vi "EventListener.vi"() -> ()   [LabVIEW 2009]
uses:
  <vilib>/lvdsc/NI_DSC.lvlib
panel:
  in  "TERMINATE MEASUREMENT":bool
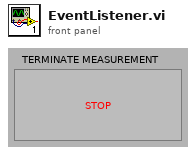
[diagram p1: front panel]
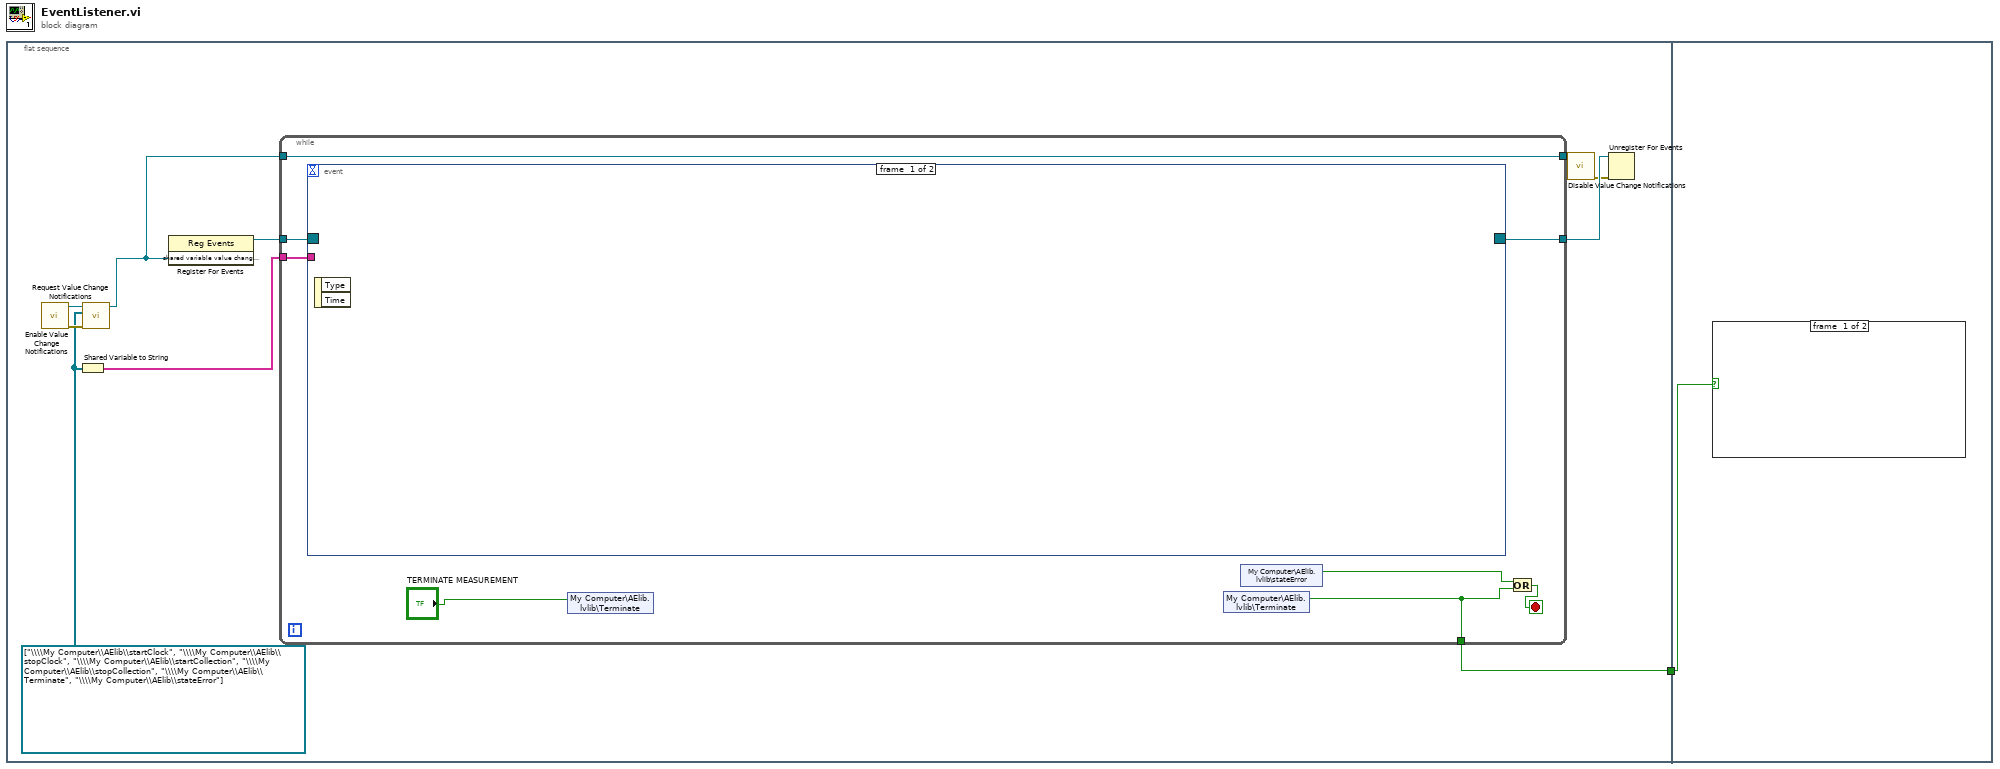
[diagram p0: block diagram]
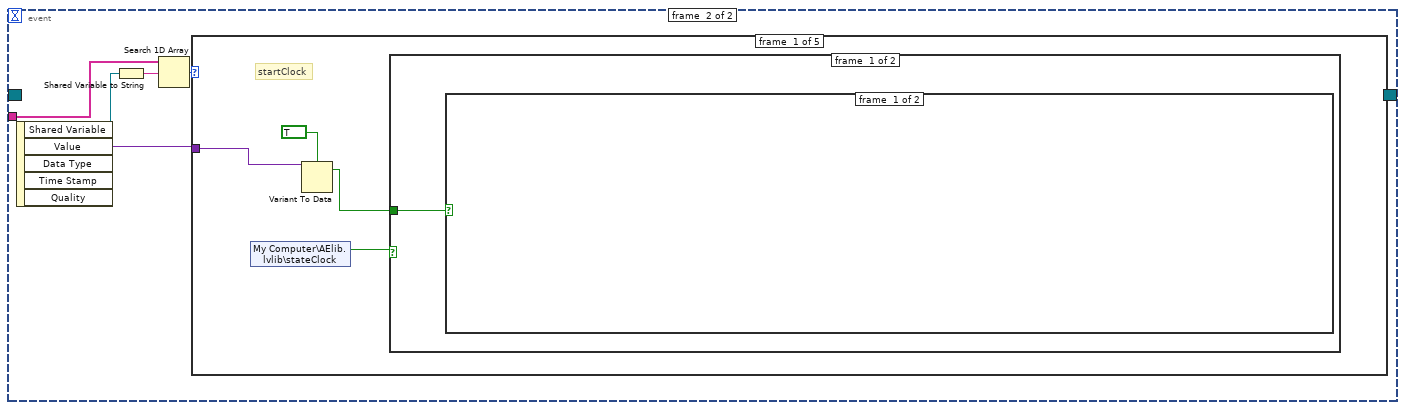
[diagram p2: hidden frame]
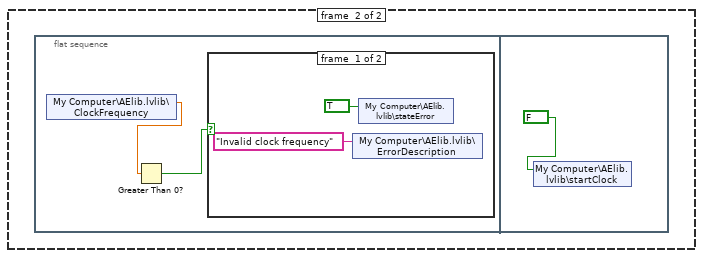
[diagram p3: hidden frame]
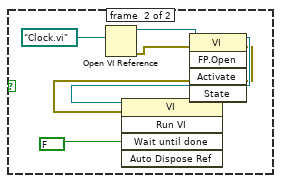
[diagram p4: hidden frame]
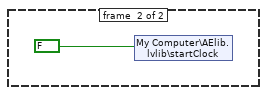
[diagram p6: hidden frame]
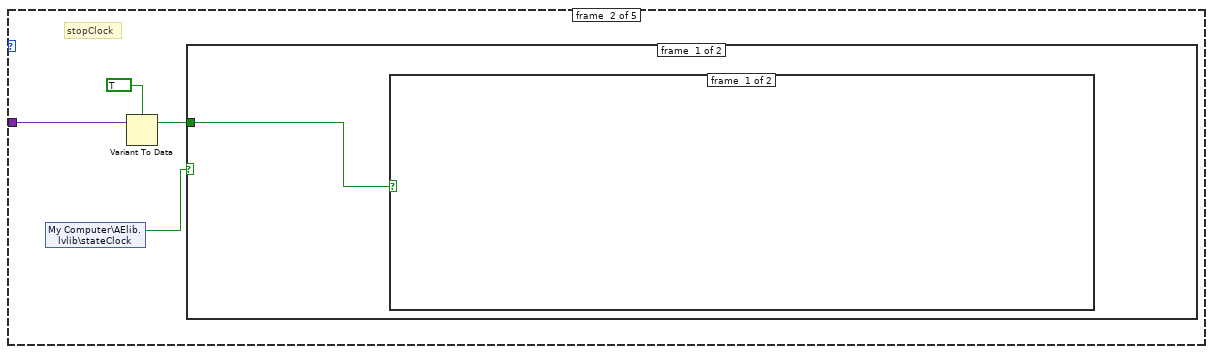
[diagram p7: hidden frame]
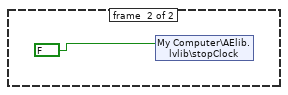
[diagram p8: hidden frame]
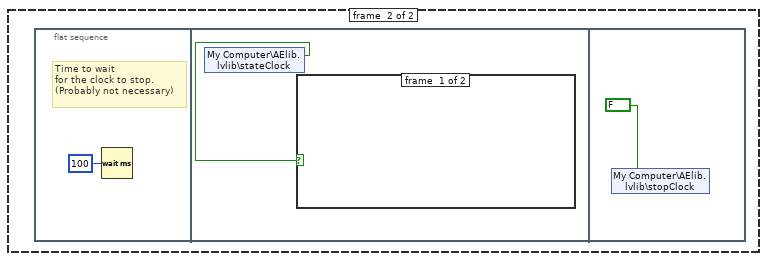
[diagram p10: hidden frame]
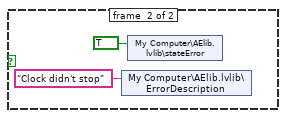
[diagram p11: hidden frame]
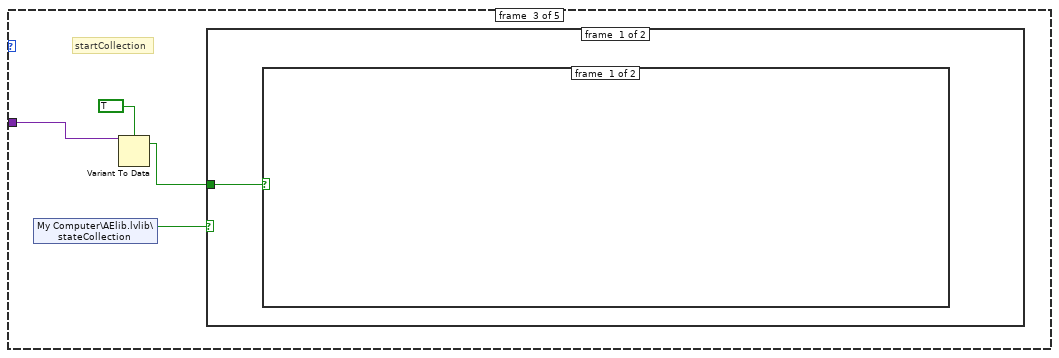
[diagram p12: hidden frame]
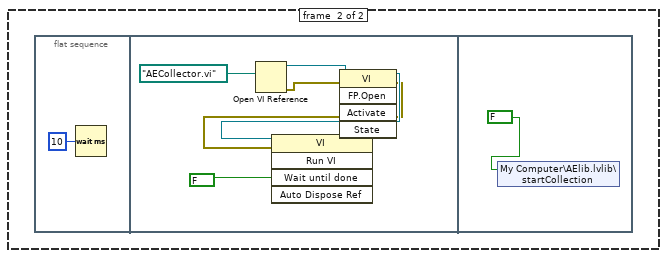
[diagram p13: hidden frame]
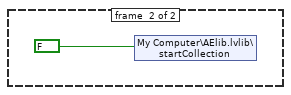
[diagram p15: hidden frame]
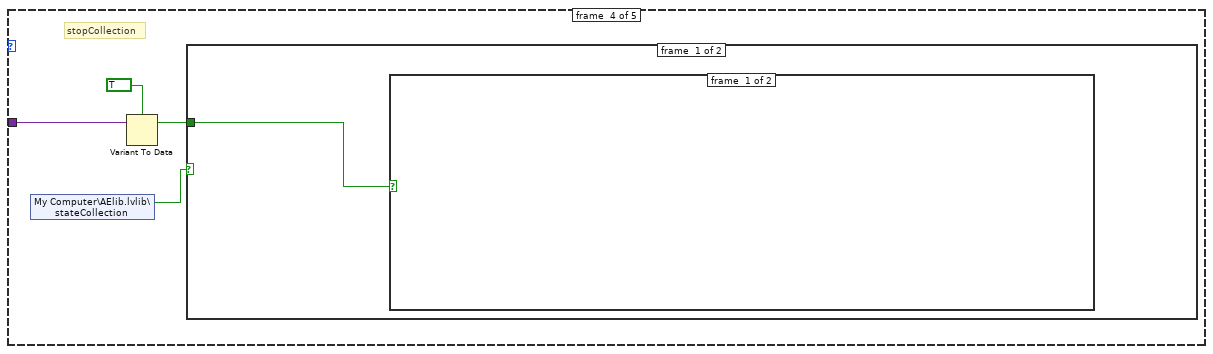
[diagram p16: hidden frame]
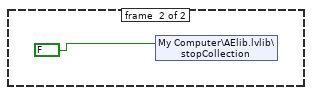
[diagram p17: hidden frame]
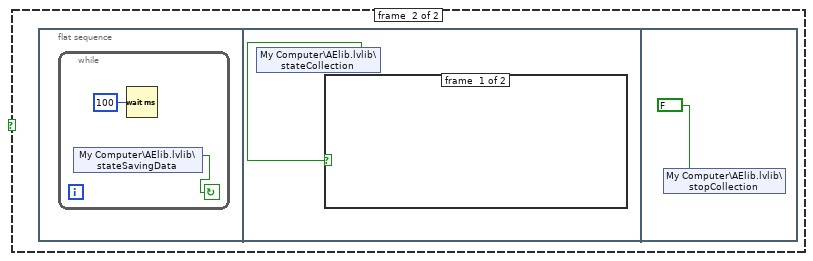
[diagram p19: hidden frame]
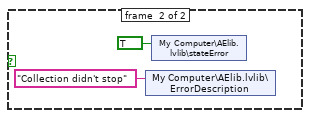
[diagram p20: hidden frame]
diagram:
  n1 = flat-sequence {
    tunnel: [w2] -> w1
    tunnel: w1 -> [w83]
    frame #0 {
      w4 = refnum<k21>[] ["\\\\My Computer\\AElib\\startClock", "\\\\My Computer\\AElib\\stopClock", "\\\\My Computer\\AElib\\startCollection", "\\\\My Computer\\AElib\\stopCollection", "\\\\My Computer\\AElib\\Terminate", "\\\\My Computer\\AElib\\stateError"] ("shared variables")
      n2 = call <vilib>:"Enable Value Change Notifications.vi"() -> ("error out"=w11:errorcluster, "shared variable value change notification"=w10:refnum<user-event>)  [unwired: 10 in]
      n3 = Shared Variable to String(1:w4) -> (0:w3:string[])
      n4 = call <vilib>:"Request Value Change Notifications.vi"("error in (no error)"=w11, "shared variables"=w4, "notification refnum"=w10) -> ("shared variable value change notification"=w8:refnum<user-event>)  [unwired: 6 in, 2 out]
      n5 = register-events(w8) -> (reference out=w9:refnum<event-registration>)  [unwired: 2 in, 1 out]
      n6 = while {
        tunnel: w9 -> [w19]
        tunnel: w8 -> [w18]
        tunnel: [w18] -> w7
        tunnel: [w17] -> w6
        tunnel: w3 -> [w16]
        tunnel: [w13] -> w2
        stop <- w14 stop-if-true
        n7 = event shown="[1] <shared variable value change notification>: User Event" {
          selector: w19 -> [_ _]
          dyn-events: [_ _] -> w17
          timeout: _ -> [_ _]
          tunnel: w16 -> [_ w22]
          event #0 {
            n8 = event-data() -> ()  [unwired: 1 in, 2 out]
          }
          event #1 {
            n9 = event-data() -> ("Shared Variable"=w24:refnum<k21>, "Value"=w20:variant)  [unwired: 1 in, 3 out]
            n10 = Shared Variable to String(1:w24) -> (0:w23:string)
            n11 = Search 1D Array(1D array=w22, element=w23) -> (index of element=w21:i32)  [unwired: 1 in]
            n12 = case shown="2" w21 {
              tunnel: w20 -> [w27 w44 w57 w71 _]
              frame #0 {
                # "startClock"
                n13 = shared-variable "My Computer\\AElib.lvlib\\stateClock"() -> (w25:bool)  [unwired: 1 in, 1 out]
                n14 = Variant To Data(Variant=w27, type=TRUE) -> (data=w26:bool)  [unwired: 1 in, 1 out]
                n15 = case shown="False" w25 {
                  tunnel: w26 -> [w29 w41]
                  frame #0 {
                    n16 = case shown="True" w29 {
                      frame #0 {
                      }
                      frame #1 {
                        n17 = flat-sequence {
                          frame #0 {
                            n18 = shared-variable "My Computer\\AElib.lvlib\\ClockFrequency"() -> (w31:dbl)  [unwired: 1 in, 1 out]
                            n19 = Greater Than 0?(x=w31) -> (x > 0?=w30:bool)
                            n20 = case shown="True" w30 {
                              frame #0 {
                                n21 = shared-variable "My Computer\\AElib.lvlib\\ErrorDescription"("Invalid clock frequency" ("ErrorDescription")) -> ()  [unwired: 1 in, 1 out]
                                n22 = shared-variable "My Computer\\AElib.lvlib\\stateError"(TRUE ("stateError")) -> ()  [unwired: 1 in, 1 out]
                              }
                              frame #1 {
                                n23 = Open VI Reference(vi path=path "Clock.vi") -> (vi reference=w37:refnum<vi>, error out=w38:errorcluster)  [unwired: 5 in]
                                n24 = invoke class="VI" method="FP.Open"(reference=w37, error in=w38) -> (reference out=w36:refnum<vi>, error out=w35:errorcluster)  [unwired: 3 in, 3 out]
                                n25 = invoke class="VI" method="Run VI"(reference=w36, error in=w35, "Wait until done"=FALSE) -> ()  [unwired: 2 in, 5 out]
                              }
                            }
                          }
                          frame #1 {
                            n26 = shared-variable "My Computer\\AElib.lvlib\\startClock"(FALSE) -> ()  [unwired: 1 in, 1 out]
                          }
                        }
                      }
                    }
                  }
                  frame #1 {
                    n27 = case shown="True" w41 {
                      frame #0 {
                      }
                      frame #1 {
                        n28 = shared-variable "My Computer\\AElib.lvlib\\startClock"(FALSE) -> ()  [unwired: 1 in, 1 out]
                      }
                    }
                  }
                }
              }
              frame #1 {
                # "stopClock"
                n29 = shared-variable "My Computer\\AElib.lvlib\\stateClock"() -> (w43:bool)  [unwired: 1 in, 1 out]
                n30 = Variant To Data(Variant=w44, type=TRUE) -> (data=w45:bool)  [unwired: 1 in, 1 out]
                n31 = case shown="True" w43 {
                  tunnel: w45 -> [w47 w49]
                  frame #0 {
                    n32 = case shown="True" w47 {
                      frame #0 {
                      }
                      frame #1 {
                        n33 = shared-variable "My Computer\\AElib.lvlib\\stopClock"(FALSE) -> ()  [unwired: 1 in, 1 out]
                      }
                    }
                  }
                  frame #1 {
                    n34 = case shown="True" w49 {
                      frame #0 {
                      }
                      frame #1 {
                        n35 = flat-sequence {
                          frame #0 {
                            # "Time to wait \nfor the clock to stop. \n(Probably not necessary)"
                            n36 = Wait (ms)(milliseconds to wait=u32 100) -> ()  [unwired: 1 out]
                          }
                          frame #1 {
                            n37 = shared-variable "My Computer\\AElib.lvlib\\stateClock"() -> (w51:bool)  [unwired: 1 in, 1 out]
                            n38 = case shown="False" w51 {
                              frame #0 {
                              }
                              frame #1 {
                                n39 = shared-variable "My Computer\\AElib.lvlib\\ErrorDescription"("Clock didn't stop" ("ErrorDescription")) -> ()  [unwired: 1 in, 1 out]
                                n40 = shared-variable "My Computer\\AElib.lvlib\\stateError"(TRUE ("stateError")) -> ()  [unwired: 1 in, 1 out]
                              }
                            }
                          }
                          frame #2 {
                            n41 = shared-variable "My Computer\\AElib.lvlib\\stopClock"(FALSE) -> ()  [unwired: 1 in, 1 out]
                          }
                        }
                      }
                    }
                  }
                }
              }
              frame #2 {
                # "startCollection"
                n42 = shared-variable "My Computer\\AElib.lvlib\\stateCollection"() -> (w55:bool)  [unwired: 1 in, 1 out]
                n43 = Variant To Data(Variant=w57, type=TRUE) -> (data=w56:bool)  [unwired: 1 in, 1 out]
                n44 = case shown="False" w55 {
                  tunnel: w56 -> [w59 w68]
                  frame #0 {
                    n45 = case shown="True" w59 {
                      frame #0 {
                      }
                      frame #1 {
                        n46 = flat-sequence {
                          frame #0 {
                            n47 = Wait (ms)(milliseconds to wait=u32 10) -> ()  [unwired: 1 out]
                          }
                          frame #1 {
                            n48 = Open VI Reference(vi path=path "AECollector.vi") -> (vi reference=w64:refnum<vi>, error out=w65:errorcluster)  [unwired: 5 in]
                            n49 = invoke class="VI" method="FP.Open"(reference=w64, error in=w65) -> (reference out=w63:refnum<vi>, error out=w62:errorcluster)  [unwired: 3 in, 3 out]
                            n50 = invoke class="VI" method="Run VI"(reference=w63, error in=w62, "Wait until done"=FALSE) -> ()  [unwired: 2 in, 5 out]
                          }
                          frame #2 {
                            n51 = shared-variable "My Computer\\AElib.lvlib\\startCollection"(FALSE) -> ()  [unwired: 1 in, 1 out]
                          }
                        }
                      }
                    }
                  }
                  frame #1 {
                    n52 = case shown="True" w68 {
                      frame #0 {
                      }
                      frame #1 {
                        n53 = shared-variable "My Computer\\AElib.lvlib\\startCollection"(FALSE) -> ()  [unwired: 1 in, 1 out]
                      }
                    }
                  }
                }
              }
              frame #3 {
                # "stopCollection"
                n54 = shared-variable "My Computer\\AElib.lvlib\\stateCollection"() -> (w70:bool)  [unwired: 1 in, 1 out]
                n55 = Variant To Data(Variant=w71, type=TRUE) -> (data=w72:bool)  [unwired: 1 in, 1 out]
                n56 = case shown="True" w70 {
                  tunnel: w72 -> [w74 w76]
                  frame #0 {
                    n57 = case shown="True" w74 {
                      frame #0 {
                      }
                      frame #1 {
                        n58 = shared-variable "My Computer\\AElib.lvlib\\stopCollection"(FALSE) -> ()  [unwired: 1 in, 1 out]
                      }
                    }
                  }
                  frame #1 {
                    n59 = case shown="True" w76 {
                      frame #0 {
                      }
                      frame #1 {
                        n60 = flat-sequence {
                          frame #0 {
                            n61 = while {
                              stop <- w78 continue-if-true
                              n62 = shared-variable "My Computer\\AElib.lvlib\\stateSavingData"() -> (w78:bool)  [unwired: 1 in, 1 out]
                              n63 = Wait (ms)(milliseconds to wait=u32 100) -> ()  [unwired: 1 out]
                            }
                          }
                          frame #1 {
                            n64 = shared-variable "My Computer\\AElib.lvlib\\stateCollection"() -> (w79:bool)  [unwired: 1 in, 1 out]
                            n65 = case shown="True" w79 {
                              frame #0 {
                              }
                              frame #1 {
                                n66 = shared-variable "My Computer\\AElib.lvlib\\ErrorDescription"("Collection didn't stop" ("ErrorDescription")) -> ()  [unwired: 1 in, 1 out]
                                n67 = shared-variable "My Computer\\AElib.lvlib\\stateError"(TRUE ("stateError")) -> ()  [unwired: 1 in, 1 out]
                              }
                            }
                          }
                          frame #2 {
                            n68 = shared-variable "My Computer\\AElib.lvlib\\stopCollection"(FALSE) -> ()  [unwired: 1 in, 1 out]
                          }
                        }
                      }
                    }
                  }
                }
              }
              frame #4 {
              }
            }
          }
        }
        n69 = shared-variable "My Computer\\AElib.lvlib\\Terminate"("TERMINATE MEASUREMENT") -> ()  [unwired: 1 in, 1 out]
        n70 = shared-variable "My Computer\\AElib.lvlib\\Terminate"() -> (w13:bool)  [unwired: 1 in, 1 out]
        n71 = shared-variable "My Computer\\AElib.lvlib\\stateError"() -> (w15:bool)  [unwired: 1 in, 1 out]
        n72 = Or(x=w15, y=w13) -> (x .or. y?=w14:bool)
      }
      n73 = call <vilib>:"Disable Value Change Notifications.vi"("notification refnum"=w7) -> ("error out"=w5:errorcluster)  [unwired: 10 in]
      n74 = Unregister For Events(event registration refnum=w6, error in=w5) -> ()  [unwired: 1 out]
    }
    frame #1 {
      n75 = case shown="True" w83 {
        frame #0 {
        }
        frame #1 {
          n76 = shared-variable "My Computer\\AElib.lvlib\\ErrorDescription"("Process terminated" ("ErrorDescription")) -> ()  [unwired: 1 in, 1 out]
          n77 = shared-variable "My Computer\\AElib.lvlib\\stateError"(TRUE ("stateError")) -> ()  [unwired: 1 in, 1 out]
        }
      }
    }
  }
